vi "Read Value.vi"(8 "error in (no error)":errorcluster caption="entrée d'erreur (pas d'erreur)", 11 "DAQmxTaskAICurrent en entrée":refnum<class "DAQmxTaskAICurrent.lvclass">) -> (0 "error out":errorcluster caption="sortie d'erreur", 1 "Data":bool, 2 "Data string":string, 3 "DAQmxTaskAICurrent en sortie":refnum<class "DAQmxTaskAICurrent.lvclass">)   [LabVIEW 2015, in "DAQmxTaskAICurrent.lvclass"]
uses:
  DAQmxTaskAICurrent.lvclass
  DAQmxTask.lvclass/DAQmxTask.ctl
  <vilib>/DAQmx/read.llb/DAQmx Read (Analog 1D DBL 1Chan NSamp).vi
  <vilib>/DAQmx/miscellaneous.llb/DAQmx Fill In Error Info.vi
  DAQmxTask.lvclass
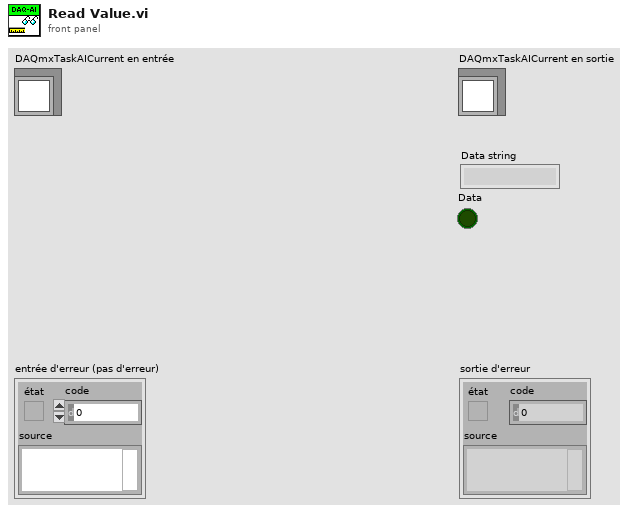
[diagram p1: front panel]
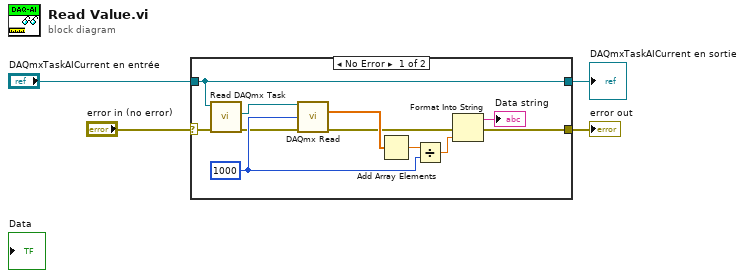
[diagram p0: block diagram]
diagram:
  n1 = case shown="No Error" "error in (no error)" {
    selector: "error in (no error)" -> [w15 w17]
    tunnel: [w8 w17] -> w1
    tunnel: [w14 w16] -> w3
    tunnel: "DAQmxTaskAICurrent en entrée" -> [w14 w16]
    frame No Error {
      w13 = 1000 ("number of samples per channel")
      n2 = call "Read DAQmx Task.vi"("error in (no error)"=w15, "DAQmxTask in"=w14) -> ("error out"=w6:errorcluster, "DAQmx Task Name"=w5:refnum<k21>)  [unwired: 7 in, 1 out]
      n3 = call-poly <vilib>:"DAQmx Read.vi"("task/channels in"=w5, "number of samples per channel"=w13, "error in"=w6) -> ("data"=w12:dbl[], "error out"=w9:errorcluster)  [unwired: 10 in, 1 out]
      n4 = Add Array Elements(numeric array=w12) -> (sum=w11:dbl)
      n5 = Divide(x=w11, y=w13) -> (x/y=w10:dbl)
      n6 = Format Into String(error in=w9, w10) -> (resulting string=→"Data string":string, error out=w8:errorcluster)  [unwired: 2 in]
    }
    frame Error {
    }
  }
  "error out" <- w1
  "DAQmxTaskAICurrent en sortie" <- w3
